vi "base64-encode.vi"(0 "binary input":string) -> (1 "base64 string":string, 2 "return code":i32)   [LabVIEW 2013]
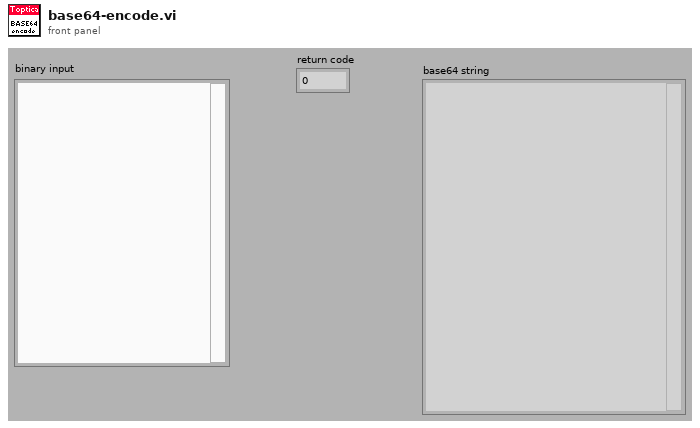
[diagram p1: front panel]
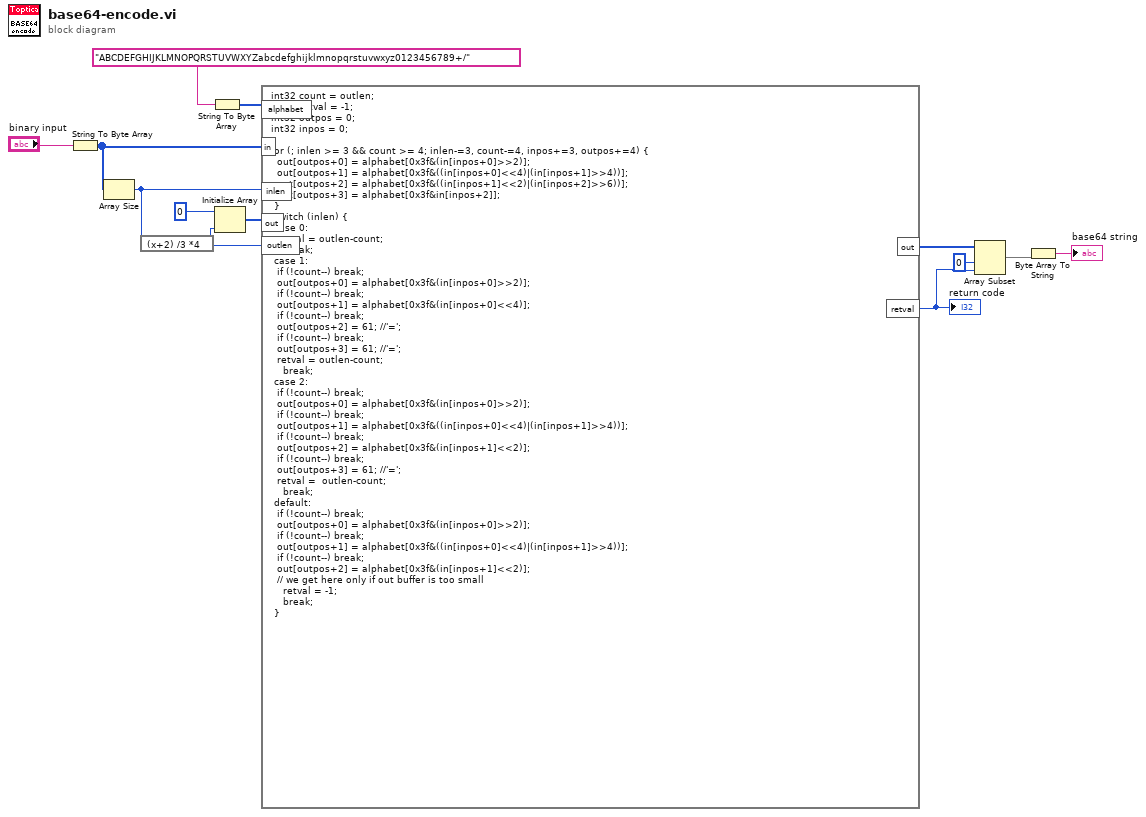
[diagram p0: block diagram]
diagram:
  n1 = String To Byte Array(string="binary input") -> (unsigned byte array=w11:u8[])
  n2 = Array Size(array=w11) -> (size(s)=w5:i32)
  n3 = expression code="(x+2) /3 *4"(w5) -> (w2:i32)
  n4 = String To Byte Array(string="ABCDEFGHIJKLMNOPQRSTUVWXYZabcdefghijklmnopqrstuvwxyz0123456789+/") -> (unsigned byte array=w13:u8[])
  n5 = Initialize Array(u8 0, w2) -> (w3:u8[])
  n6 = formula code="int32 count = outlen;\nint32 retval = -1;\nint32 outpos = 0;\nint32 inpos = 0;\n\nfor (; inlen >= 3 && count >= 4; inlen-=3, count-=4, inpos+=3, outpos+=4) {\n\t\tout[outpos+0] = alphabet[0x3f&(in[inpos+0]>>2)];\n\t\tout[outpos+1] = alphabet[0x3f&((in[inpos+0]<<4)|(in[inpos+1]>>4))];\n\t\tout[outpos+2] = alphabet[0x3f&((in[inpos+1]<<2)|(in[inpos+2]>>6))];\n\t\tout[outpos+3] = alphabet[0x3f&in[inpos+2]];\n\t}\n\tswitch (inlen) {\n\tcase 0:\n\t\tretval = outlen-count;\n    break;\n\tcase 1:\n\t\tif (!count--) break;\n\t\tout[outpos+0] = alphabet[0x3f&(in[inpos+0]>>2)];\n\t\tif (!count--) break;\n\t\tout[outpos+1] = alphabet[0x3f&(in[inpos+0]<<4)];\n\t\tif (!count--) break;\n\t\tout[outpos+2] = 61; //'=';\n\t\tif (!count--) break;\n\t\tout[outpos+3] = 61; //'=';\n\t\tretval = outlen-count;\n    break;\n\tcase 2:\n\t\tif (!count--) break;\n\t\tout[outpos+0] = alphabet[0x3f&(in[inpos+0]>>2)];\n\t\tif (!count--) break;\n\t\tout[outpos+1] = alphabet[0x3f&((in[inpos+0]<<4)|(in[inpos+1]>>4))];\n\t\tif (!count--) break;\n\t\tout[outpos+2] = alphabet[0x3f&(in[inpos+1]<<2)];\n\t\tif (!count--) break;\n\t\tout[outpos+3] = 61; //'=';\n\t\tretval =  outlen-count;\n    break;\n\tdefault:\n\t\tif (!count--) break;\n\t\tout[outpos+0] = alphabet[0x3f&(in[inpos+0]>>2)];\n\t\tif (!count--) break;\n\t\tout[outpos+1] = alphabet[0x3f&((in[inpos+0]<<4)|(in[inpos+1]>>4))];\n\t\tif (!count--) break;\n\t\tout[outpos+2] = alphabet[0x3f&(in[inpos+1]<<2)];\n\t\t// we get here only if out buffer is too small\n    retval = -1;\n    break;\n\t}"("in"=w11, "alphabet"=w13, "inlen"=w5, "out"=w3, "outlen"=w2) -> ("out"=w10:u8[], "retval"=w1:i32)
  "return code" <- w1
  n7 = Array Subset(array=w10, index=0, length=w1) -> (w8:u8[])
  n8 = Byte Array To String(unsigned byte array=w8) -> (string=→"base64 string":string)
